vi "BuildMenu.vi"(0 "XRef":T7, 1 "MenuRef":T6, 2 "Point":T4, 3 "Menu Type":T3, 4 "State In":T2) -> (14 "Fatal Error Out":T1)   [LabVIEW 2015, in "LVJSON.lvlib" / "Get Object Parameters.xnode"]
uses:
  Get Object Parameters.xnode
  <vilib>/XNodeSupport/XNodeXNodeRef.ctl
  <vilib>/XNodeSupport/XNodeMenuRef.ctl
  <vilib>/XNodeSupport/XNodePoint.ctl
  <vilib>/XNodeSupport/XNodeInt.ctl
  <vilib>/XNodeSupport/XNodeMenuType.ctl
  State.ctl
  <vilib>/XNodeSupport/XNodeErrorCluster.ctl
  dimensions.vi
  <vilib>/XNodeSupport/NI_XNodeSupport.lvlib
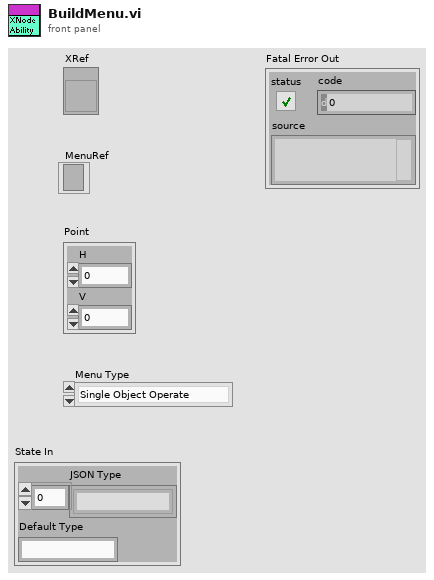
[diagram p1: front panel]
types:
  T1 = typedef "NI_XNodeSupport.lvlib/XNodeErrorCluster.ctl" = errorcluster
  T2 = typedef "LVJSON.lvlib/Get Object Parameters.xnode/State.ctl" = cluster{"JSON Type":string[], "Default Type":string}
  T3 = typedef "NI_XNodeSupport.lvlib/XNodeMenuType.ctl" = enum32{"Single Object Operate", "Single Object Popup", "Multi Object Popup Master", "Multi Object Popup Other"}
  T4 = typedef "NI_XNodeSupport.lvlib/XNodePoint.ctl" = cluster{"H":T5, "V":T5}
  T5 = typedef "NI_XNodeSupport.lvlib/XNodeInt.ctl" = i32
  T6 = typedef "NI_XNodeSupport.lvlib/XNodeMenuRef.ctl" = refnum<k9>
  T7 = typedef "NI_XNodeSupport.lvlib/XNodeXNodeRef.ctl" = refnum<vi>
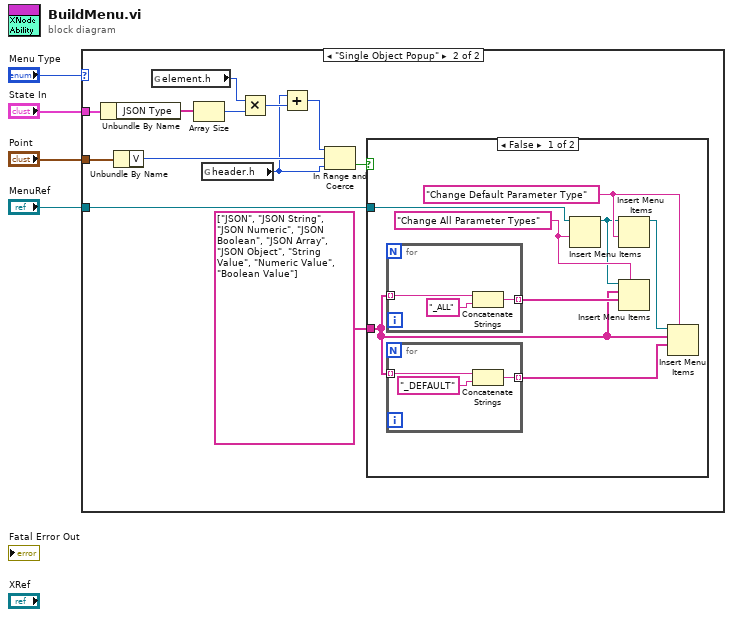
[diagram p0: block diagram]
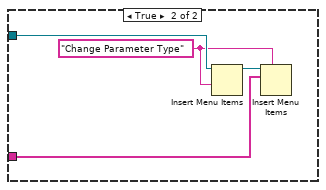
[diagram p3: hidden frame]
diagram:
  n1 = case shown="\"Single Object Popup\"" "Menu Type" {
    tunnel: "MenuRef" -> [_ w16]
    tunnel: "Point" -> [_ w15]
    tunnel: "State In" -> [_ w14]
    frame "Single Object Operate", Default {
    }
    frame "Single Object Popup" {
      n2 = Unbundle By Name(w14) -> ("JSON Type"=w7:string[])
      n3 = Unbundle By Name(w15) -> ("V"=w10:T5)
      n4 = global read "dimensions.vi" "element.h"() -> (w13:i16)
      n5 = Array Size(array=w7) -> (size(s)=w6:i32)
      n6 = global read "dimensions.vi" "header.h"() -> (w8:i16)
      n7 = Multiply(x=w13, y=w6) -> (x*y=w12:i32)
      n8 = Add(x=w8, y=w12) -> (x+y=w9:i32)
      n9 = In Range and Coerce(upper limit=w9, x=w10, lower limit=w8) -> (In Range?=w11:bool)  [unwired: 1 out]
      n10 = case shown="False" w11 {
        tunnel: w16 -> [w24 w34]
        tunnel: string[] ["JSON", "JSON String", "JSON Numeric", "JSON Boolean", "JSON Array", "JSON Object", "String Value", "Numeric Value", "Boolean Value"] ("item names") -> [w17 w31]
        frame False {
          w20 = "Change Default Parameter Type" ("menu tag")
          w23 = "Change All Parameter Types" ("menu tag")
          n11 = for {
            tunnel: w17 -> [w30] mode=indexing
            tunnel: [w28] -> w22 mode=indexing
            n12 = Concatenate Strings(w30, "_ALL" ("string")) -> (w28:string)
          }
          n13 = for {
            tunnel: w17 -> [w27] mode=indexing
            tunnel: [w25] -> w21 mode=indexing
            n14 = Concatenate Strings(w27, "_DEFAULT" ("string")) -> (w25:string)
          }
          n15 = Insert Menu Items(7:w23, 9:w24) -> (3:w18:refnum<k9>)  [unwired: 4 in, 2 out]
          n16 = Insert Menu Items(7:w20, 9:w18) -> (3:w19:refnum<k9>)  [unwired: 4 in, 2 out]
          n17 = Insert Menu Items(5:w23, 7:w22, 8:w17, 9:w18) -> ()  [unwired: 2 in, 3 out]
          n18 = Insert Menu Items(5:w20, 7:w21, 8:w17, 9:w19) -> ()  [unwired: 2 in, 3 out]
        }
        frame True {
          w32 = "Change Parameter Type"
          n19 = Insert Menu Items(7:w32, 9:w34) -> (3:w33:refnum<k9>)  [unwired: 4 in, 2 out]
          n20 = Insert Menu Items(5:w32, 8:w31, 9:w33) -> ()  [unwired: 3 in, 3 out]
        }
      }
    }
  }
